vi "sub parse frame i.vi"(8 "error in (no error)":errorcluster, 11 "<i> String":string="   <i kind 6 x -4 y 21 w 85 h 65 vrest 1 i>") -> (0 "error out":errorcluster, 3 "<i> data":T1)   [LabVIEW 2018, in "Frame Analizer.lvclass"]
uses:
  Frame Analizer.lvclass
  frame i data.ctl
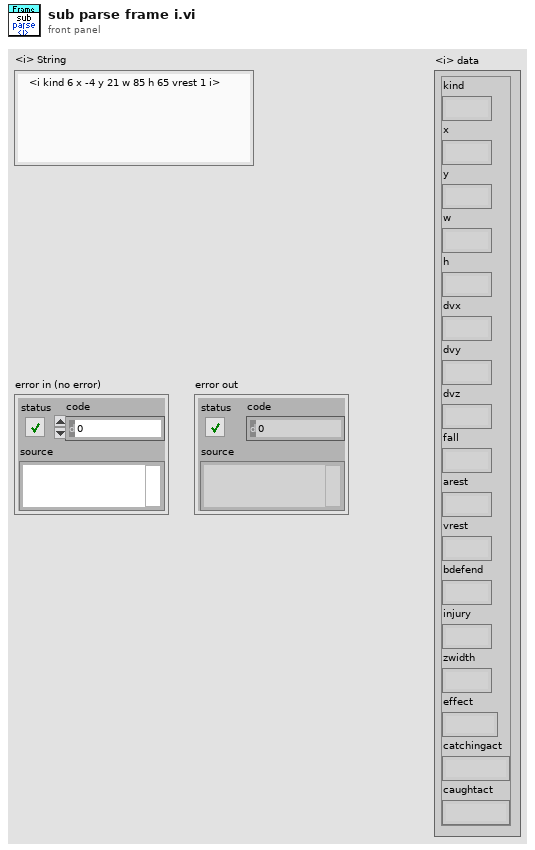
[diagram p1: front panel]
types:
  T1 = typedef "Frame Analizer.lvclass/frame i data.ctl" = cluster{"kind":string, "x":string, "y":string, "w":string, "h":string, "dvx":string, "dvy":string, "dvz":string, "fall":string, "arest":string, "vrest":string, "bdefend":string, "injury":string, "zwidth":string, "effect":string, "catchingact":string, "caughtact":string}
  T2 = cluster{"keyword":string, "value 1":string, "value 2":string}[]
  T3 = cluster{"[0]":string, "[1]":string, "[2]":string, "[3]":string, "[4]":string, "[5]":string, "[6]":string, "[7]":string, "[8]":string, "[9]":string, "[10]":string, "[11]":string, "[12]":string, "[13]":string, "[14]":string}
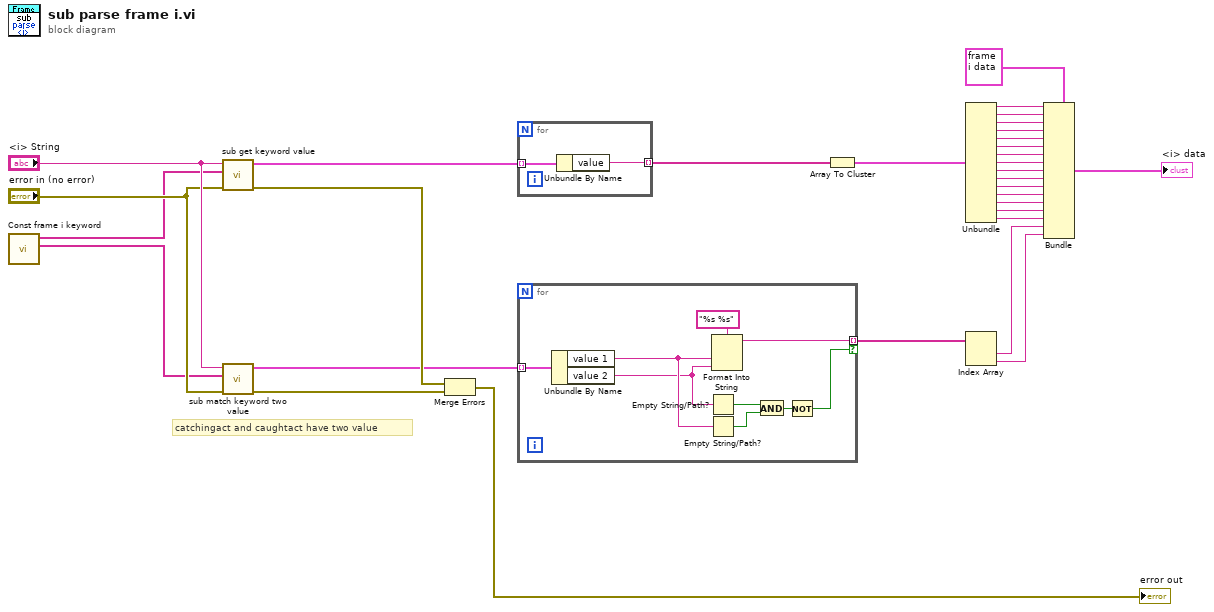
[diagram p0: block diagram]
diagram:
  # "catchingact and caughtact have two value"
  n1 = call "Const frame i keyword.vi"() -> ("Const frame i keyword 2"=w2:string[], "Const frame i keyword"=w3:string[])  [unwired: 10 in]
  n2 = call "sub get keyword value.vi"("error in"="error in (no error)", "keyword"=w3, "string"="<i> String") -> ("error out"=w7:errorcluster, "matched pairs (all)"=w31:cluster{"keyword":string, "value":string}[])  [unwired: 5 in, 2 out]
  n3 = call "sub match keyword two value.vi"("error in"="error in (no error)", "keyword"=w2, "string"="<i> String") -> ("error out"=w8:errorcluster, "matched pairs (all)"=w4:T2)  [unwired: 5 in, 2 out]
  n4 = Merge Errors(w7, w8) -> (→"error out":errorcluster)
  n5 = for {
    tunnel: w31 -> [w33] mode=indexing
    tunnel: [w32] -> w30 mode=indexing
    n6 = Unbundle By Name(w33) -> ("value"=w32:string)
  }
  n7 = for {
    tunnel: w4 -> [w42] mode=indexing
    tunnel: [w40] -> w11 mode=indexing if=w34
    n8 = Unbundle By Name(w42) -> ("value 1"=w39:string, "value 2"=w38:string)
    n9 = Empty String/Path?(string/path=w38) -> (empty?=w37:bool)
    n10 = Empty String/Path?(string/path=w39) -> (empty?=w36:bool)
    n11 = Format Into String(format string="%s %s", w39, w38) -> (resulting string=w40:string)  [unwired: 2 in, 1 out]
    n12 = And(x=w37, y=w36) -> (x .and. y?=w35:bool)
    n13 = Not(x=w35) -> (.not. x?=w34:bool)
  }
  n14 = Array To Cluster(array=w30) -> (cluster=w28:T3)
  n15 = Unbundle(w28) -> ("[0]"=w25:string, "[1]"=w24:string, "[2]"=w23:string, "[3]"=w22:string, "[4]"=w21:string, "[5]"=w20:string, "[6]"=w19:string, "[7]"=w18:string, "[8]"=w17:string, "[9]"=w16:string, "[10]"=w15:string, "[11]"=w14:string, "[12]"=w13:string, "[13]"=w12:string, "[14]"=w1:string)
  n16 = Index Array(array=w11) -> (element #1=w10:string, element #2=w9:string)  [unwired: 2 in]
  n17 = Bundle(cluster=T1 {"kind"="", "x"="", "y"="", "w"="", "h"="", "dvx"="", "dvy"="", "dvz"="", "fall"="", "arest"="", "vrest"="", "bdefend"="", "injury"="", "zwidth"="", "effect"="", "catchingact"="", "caughtact"=""} ("<i> data 2"), "kind"=w25, "x"=w24, "y"=w23, "w"=w22, "h"=w21, "dvx"=w20, "dvy"=w19, "dvz"=w18, "fall"=w17, "arest"=w16, "vrest"=w15, "bdefend"=w14, "injury"=w13, "zwidth"=w12, "effect"=w1, "catchingact"=w10, "caughtact"=w9) -> (→"<i> data":T1)
